vi "increment_hole_progress.vi"(8 "error in":errorcluster) -> (0 "error out":errorcluster)   [LabVIEW 2018]
uses:
  MainFGV/modes_mains_FGV.ctl
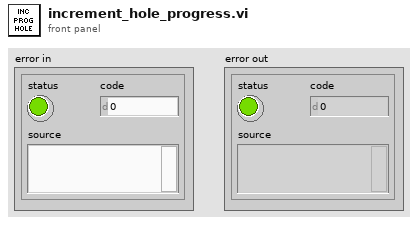
[diagram p1: front panel]
types:
  T1 = typedef "modes_mains_FGV.ctl" = enum16{"Init", "Config", "CreateDir", "CreateTask", "CreateQueues", "Record", "Comment", "GetFeed", "GetInc", "End"}
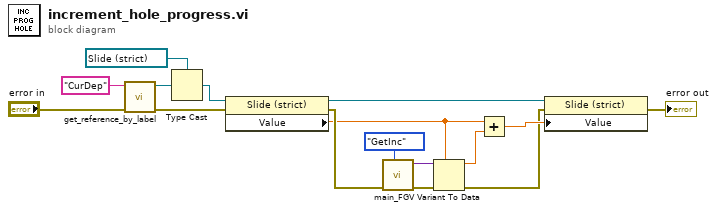
[diagram p0: block diagram]
diagram:
  n1 = call "get_reference_by_label.vi"("error in"="error in", "Label"="CurDep") -> ("error out"=w11:errorcluster, "Ctl Refnum"=w8:refnum<vi>)  [unwired: 7 in, 1 out]
  n2 = Type Cast(type=refnum<vi> refnum ("CurDep"), x=w8) -> (*(type *) &x=w10:refnum<vi>)
  n3 = property on="Property Node" class="Slide (strict)"(reference=w10, error in=w11) -> (reference out=w14:refnum<vi>, error out=w13:errorcluster, "Value"=w12:dbl)
  n4 = call "main_FGV.vi"("Mode"=modes_mains_FGV."GetInc", "error in"=w13) -> ("error out"=w4:errorcluster, "Parameter out"=w5:variant)  [unwired: 8 in]
  n5 = Variant To Data(error in=w4, type=w12, Variant=w5) -> (data=w3:dbl, error out=w1:errorcluster)
  n6 = Add(x=w12, y=w3) -> (x+y=w2:dbl)
  n7 = property on="Property Node" class="Slide (strict)"(reference=w14, error in=w1, "Value"=w2) -> (error out=→"error out":errorcluster)  [unwired: 1 out]
